vi "PV HiLobe Status requests.vi"(8 "error in (no error)":errorcluster, 9 "Parameter choice":T1(ring), 10 "Adress of unit":u16=1 min=1 max=999 step=1, 11 "VISA session":refnum<visa-resource-name>) -> (0 "error out":errorcluster, 2 "response (data)":string, 3 "dup VISA session":refnum<visa-resource-name>)   [LabVIEW 2021, in "Pfeiffer Vacuum.lvlib"]
doc: "There are 14 parameters available, only one of which can be enabled at a time. \n\nError code [303]\nActual Speed (Hz) [309]\nPump operating hours (h) [311]\nSoftware version of the interface board [312]\nSupply voltage (V) [313]\nNominal speed (Hz) [315]\nDrive power (W) [316]\nDrive current (A) [317]\nTemperatur of power electronic [324]\nDevice designation [349]\nFirmware of frequency converter [352]\nHardware version of the interface board [354]\nAcutal speed (rpm) [398]\nNominal speed (rpm) [399]\n\nNote: read only VI´s"
uses:
  <instrlib>/Pfeiffer Vacuum/Pfeiffer Vacuum.lvlib
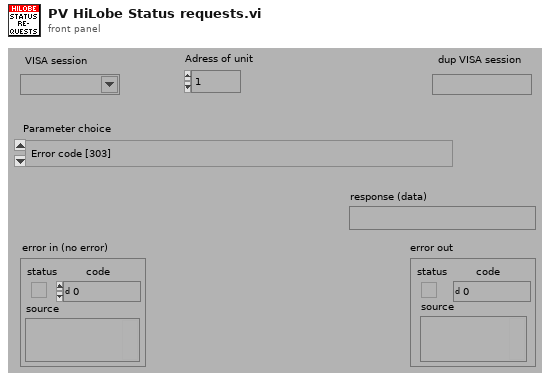
[diagram p1: front panel]
types:
  T1 = enum16{"Error code [303]", "Actual Speed (Hz) [309]", "Pump operating hours (h) [311]", "Software version of the interface board [312]", "Supply voltage (V) [313]", "Nominal speed (Hz) [315]", "Drive power (W) [316]", "Motor current (A) [317]", "Temperatur of power electronic [324]", "Device designation [349]", "Firmware of frequency converter [352]", "Hardware version of the interface board [354]", "Acutal speed (rpm) [398]", "Nominal speed (rpm) [399]"}
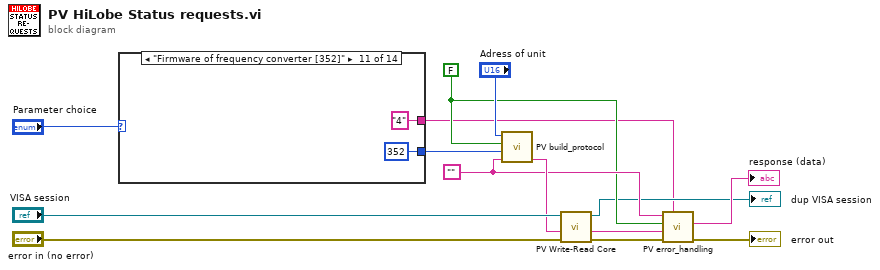
[diagram p0: block diagram]
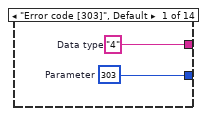
[diagram p2: hidden frame]
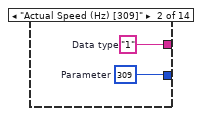
[diagram p3: hidden frame]
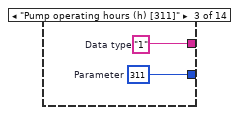
[diagram p4: hidden frame]
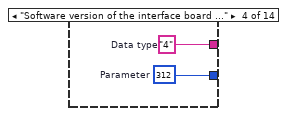
[diagram p5: hidden frame]
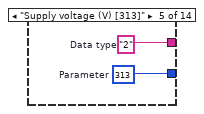
[diagram p6: hidden frame]
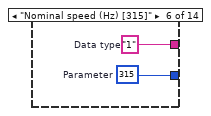
[diagram p7: hidden frame]
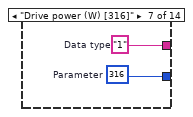
[diagram p8: hidden frame]
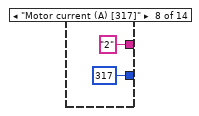
[diagram p9: hidden frame]
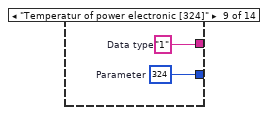
[diagram p10: hidden frame]
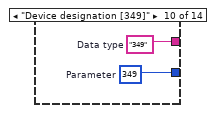
[diagram p11: hidden frame]
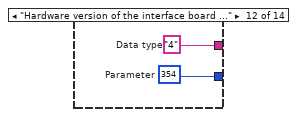
[diagram p12: hidden frame]
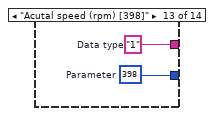
[diagram p13: hidden frame]
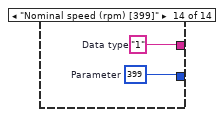
[diagram p14: hidden frame]
diagram:
  w10 = ""
  w9 = FALSE
  n1 = case shown="\"Firmware of frequency converter [352]\"" "Parameter choice" {
    tunnel: [w15 w18 w20 w22 w24 w26 w28 "2" ("Data type") w32 w34 "4" ("Data type") w38 w40 w42] -> w2
    tunnel: [w16 w17 w19 w21 w23 w25 w27 317 ("Parameter") w31 w33 352 ("Parameter") w37 w39 w41] -> w1
    frame "Error code [303]", Default {
      w15 = "4"  # Data type
      w16 = 303  # Parameter
    }
    frame "Actual Speed (Hz) [309]" {
      w17 = 309  # Parameter
      w18 = "1"  # Data type
    }
    frame "Pump operating hours (h) [311]" {
      w19 = 311  # Parameter
      w20 = "1"  # Data type
    }
    frame "Software version of the interface board [312]" {
      w21 = 312  # Parameter
      w22 = "4"  # Data type
    }
    frame "Supply voltage (V) [313]" {
      w23 = 313  # Parameter
      w24 = "2"  # Data type
    }
    frame "Nominal speed (Hz) [315]" {
      w25 = 315  # Parameter
      w26 = "1"  # Data type
    }
    frame "Drive power (W) [316]" {
      w27 = 316  # Parameter
      w28 = "1"  # Data type
    }
    frame "Motor current (A) [317]" {
    }
    frame "Temperatur of power electronic [324]" {
      w31 = 324  # Parameter
      w32 = "1"  # Data type
    }
    frame "Device designation [349]" {
      w33 = 349  # Parameter
      w34 = "349"  # Data type
    }
    frame "Firmware of frequency converter [352]" {
    }
    frame "Hardware version of the interface board [354]" {
      w37 = 354  # Parameter
      w38 = "4"  # Data type
    }
    frame "Acutal speed (rpm) [398]" {
      w39 = 398  # Parameter
      w40 = "1"  # Data type
    }
    frame "Nominal speed (rpm) [399]" {
      w41 = 399  # Parameter
      w42 = "1"  # Data type
    }
  }
  n2 = call <instrlib>:"PV build_protocol.vi"("Data"=w10, "Parameter-number"=w1, "parameter\nread<->describe"=w9, "Adress"="Adress of unit") -> ("output"=w11:string)  [unwired: 3 in]
  n3 = call <instrlib>:"PV Write-Read Core.vi"("error in"="error in (no error)", "Write data in"=w11, "VISA session"="VISA session") -> ("error out"=w7:errorcluster, "response (data) out"=w8:string, "dup VISA session"=→"dup VISA session":refnum<visa-resource-name>)  [unwired: 2 in]
  n4 = call <instrlib>:"PV error_handling.vi"("Data Typ in"=w2, "error in"=w7, "response (data) in"=w8, "Parameter\nread only<->describe"=w9, "data in"=w10) -> ("error out"=→"error out":errorcluster, "Data out"=→"response (data)":string)  [unwired: 4 in, 1 out]
